vi "macro_Cmd_Follow_RamseteExecute.vi"() -> ()   [LabVIEW 2019, in "PathPlanner24.lvlib"]
uses:
  PathPlanner24.lvlib
  <vilib>/Rock Robotics/WPI/ThirdParty/JAS_Junk/TrajLib/Trajectory_Library.lvlib
  <vilib>/Rock Robotics/WPI/ThirdParty/JAS_Junk/TrajLib/TypeDef/TRANSLATION2D.ctl
  <vilib>/Rock Robotics/WPI/ThirdParty/JAS_Junk/TrajLib/TypeDef/ROTATION2D.ctl
  <vilib>/Rock Robotics/WPI/ThirdParty/JAS_Junk/TrajLib/TypeDef/POSE2D.ctl
  TypeDef/PathPlannerPathConstraints.ctl
  TypeDef/PathPlannerRotationTarget.ctl
  TypeDef/PathPlannerConstraintsZone.ctl
  ENum/PathPlanner_CommandUtilType_ENUM.ctl
  TypeDef/PathPlannerCommandUtil.ctl
  TypeDef/PathPlannerEventMarker.ctl
  TypeDef/PathPlannerGoalEndState.ctl
  TypeDef/PathPlannerPathPoint.ctl
  TypeDef/PathPlannerPath.ctl
  <vilib>/Rock Robotics/WPI/ThirdParty/JAS_Junk/TrajLib/TypeDef/CHASSIS_SPEEDS.ctl
panel:
  out "Complete":bool
  in  "CurrentChassisSpeeds":T1 {"vOmega" format="%10.3f"; "vY" format="%10.3f"; "vX" format="%10.3f"}
  in  "PathPlannerPath":T2={"BezierPoints"=[], "PreviewStartingRotation"={"VALUE"=0.0, "COS"=1.0, "SIN"=0.0}, "Reversed"=FALSE, "RotationTargets"=[], "ConstraintZones"=[], "EventMarkers"=[], "GlobalConstraints"={"MaxVelocityMps;"=0.0, "MaxAccelerationMpsSq;"=0.0, "MaxAngularVelRadPsEc;"=0.0, "MaxAngularAccRadPSecSq"=0.0, "Exists"=FALSE, "Unlimited"=FALSE, "NominalVoltageVolts"=12.0}, "GoalEndState"={"VelocityMPS"=0.0, "Rotation"={"VALUE"=0.0, "COS"=1.0, "SIN"=0.0}}, "AllPoints"=[]} {"AllPoints"."HolonomicRotation"."SIN" format="%13.4f"; "AllPoints"."HolonomicRotation"."COS" format="%13.4f"; "AllPoints"."HolonomicRotation"."VALUE" format="%13.4f"; "AllPoints"."Position"."Y" format="%14.3f"; "AllPoints"."Position"."X" format="%14.3f"; "GoalEndState"."Rotation"."SIN" format="%13.4f"; "GoalEndState"."Rotation"."COS" format="%13.4f"; "GoalEndState"."Rotation"."VALUE" format="%13.4f"; "RotationTargets"."rotation"."SIN" format="%13.4f"; "RotationTargets"."rotation"."COS" format="%13.4f"; "RotationTargets"."rotation"."VALUE" format="%13.4f"; "PreviewStartingRotation"."SIN" format="%13.4f"; "PreviewStartingRotation"."COS" format="%13.4f"; "PreviewStartingRotation"."VALUE" format="%13.4f"; "BezierPoints"."Y" format="%14.3f"; "BezierPoints"."X" format="%14.3f"}
  out "Left Speed Dmd M/S":dbl
  out "Right Speed Dmd M/S":dbl
  in  "Reset":bool
  in  "currentPose":T13={"TRANSLATION"={"X"=0.0, "Y"=0.0}, "ROTATION"={"VALUE"=0.0, "COS"=1.0, "SIN"=0.0}} {"ROTATION"."SIN" format="%13.4f"; "ROTATION"."COS" format="%13.4f"; "ROTATION"."VALUE" format="%13.4f"; "TRANSLATION"."Y" format="%14.3f"; "TRANSLATION"."X" format="%14.3f"}
  out "Position Error M":dbl
  out "At Reference":bool
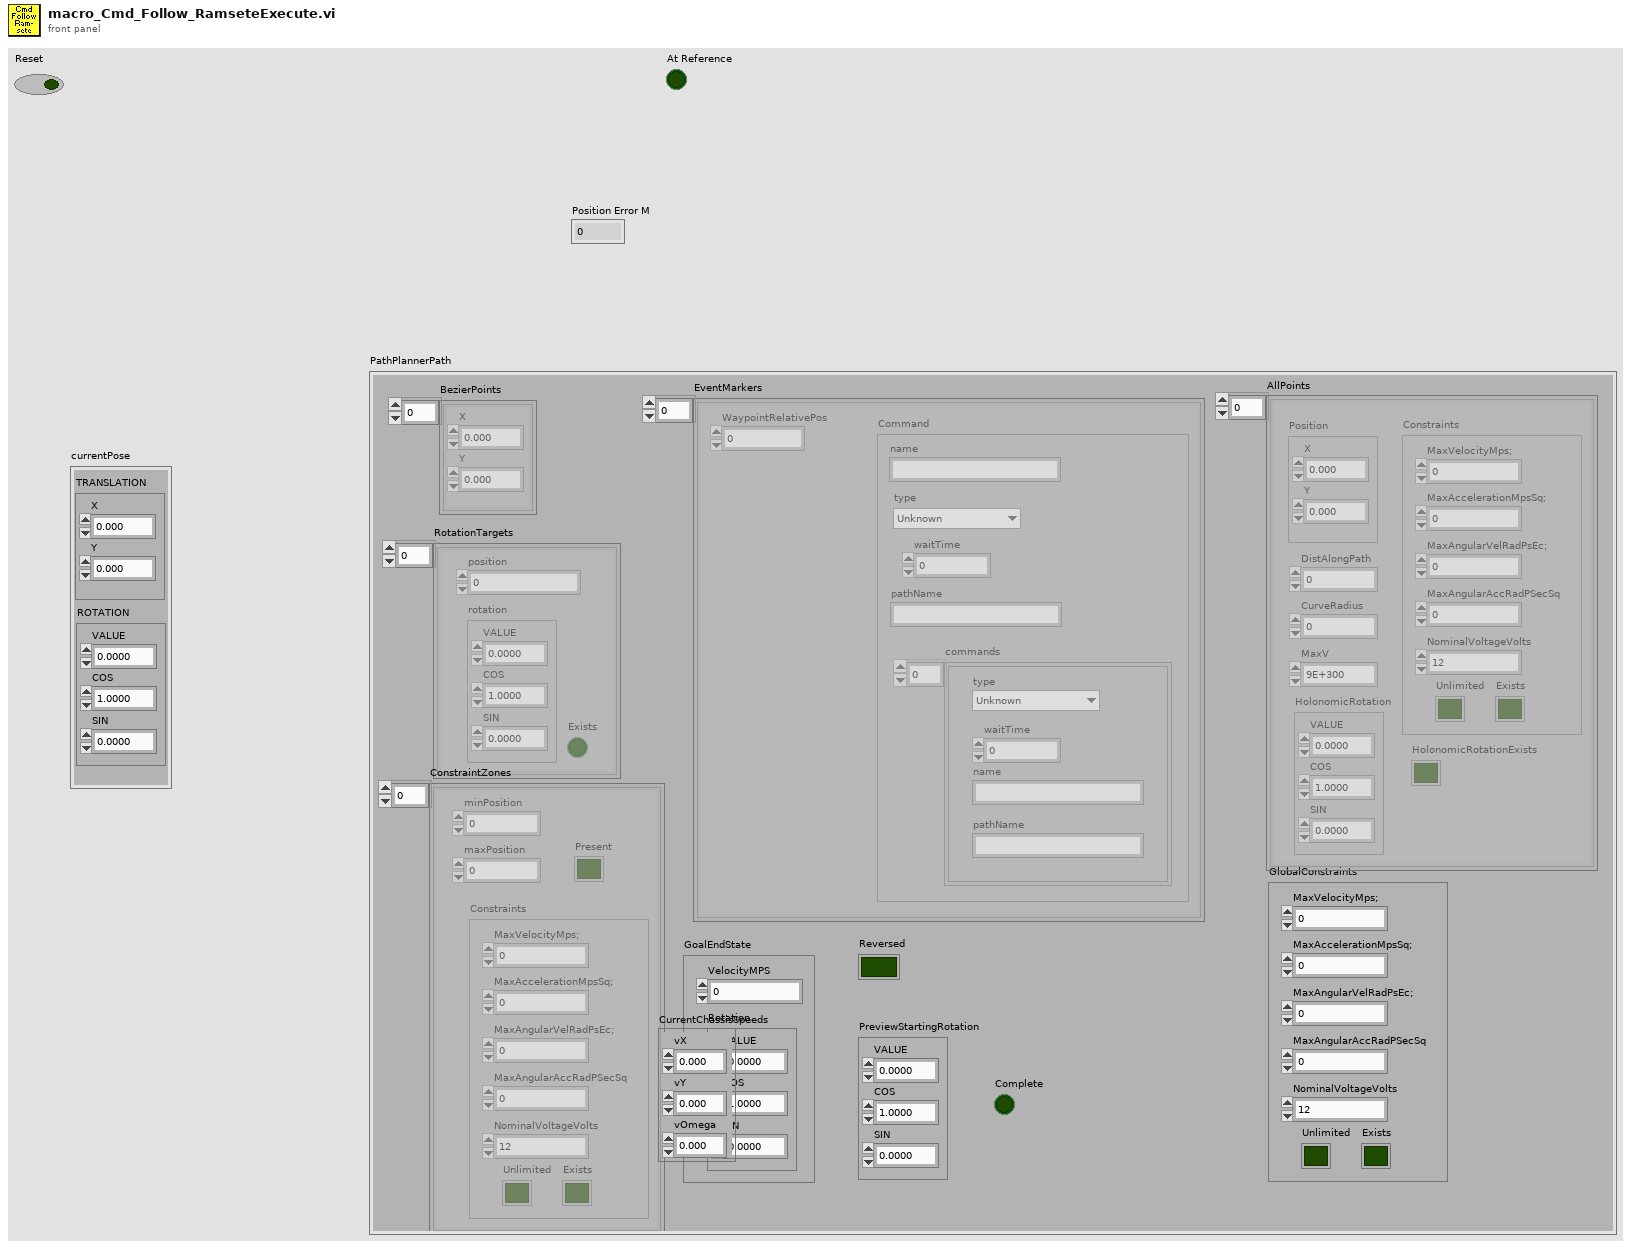
[diagram p1: front panel]
types:
  T1 = typedef "Trajectory_Library.lvlib/CHASSIS_SPEEDS.ctl" = cluster{"vX":dbl, "vY":dbl, "vOmega":dbl}
  T2 = typedef "PathPlanner24.lvlib/PathPlannerPath.ctl" = cluster{"BezierPoints":T3[], "PreviewStartingRotation":T4, "Reversed":bool, "RotationTargets":T5[], "ConstraintZones":T6[], "EventMarkers":T8[], "GlobalConstraints":T7, "GoalEndState":T11, "AllPoints":T12[]}
  T3 = typedef "Trajectory_Library.lvlib/TRANSLATION2D.ctl" = cluster{"X":dbl, "Y":dbl}
  T4 = typedef "Trajectory_Library.lvlib/ROTATION2D.ctl" = cluster{"VALUE":dbl, "COS":dbl, "SIN":dbl}
  T5 = typedef "PathPlanner24.lvlib/PathPlannerRotationTarget.ctl" = cluster{"rotation":T4, "position":dbl, "Exists":bool}
  T6 = typedef "PathPlanner24.lvlib/PathPlannerConstraintsZone.ctl" = cluster{"minPosition":dbl, "maxPosition":dbl, "Constraints":T7, "Present":bool}
  T7 = typedef "PathPlanner24.lvlib/PathPlannerPathConstraints.ctl" = cluster{"MaxVelocityMps;":dbl, "MaxAccelerationMpsSq;":dbl, "MaxAngularVelRadPsEc;":dbl, "MaxAngularAccRadPSecSq":dbl, "Exists":bool, "Unlimited":bool, "NominalVoltageVolts":dbl}
  T8 = typedef "PathPlanner24.lvlib/PathPlannerEventMarker.ctl" = cluster{"WaypointRelativePos":dbl, "Command":T9}
  T9 = typedef "PathPlanner24.lvlib/PathPlannerCommandUtil.ctl" = cluster{"waitTime":dbl, "name":string, "pathName":string, "commands":cluster{"type":T10, "waitTime":dbl, "name":string, "pathName":string}[], "type":T10}
  T10 = typedef "PathPlanner24.lvlib/PathPlanner_CommandUtilType_ENUM.ctl" = enum16{"Unknown", "Wait", "Named", "Path", "Sequential", "Parallel", "Race", "Deadline"}
  T11 = typedef "PathPlanner24.lvlib/PathPlannerGoalEndState.ctl" = cluster{"VelocityMPS":dbl, "Rotation":T4}
  T12 = typedef "PathPlanner24.lvlib/PathPlannerPathPoint.ctl" = cluster{"Position":T3, "HolonomicRotation":T4, "DistAlongPath":dbl, "CurveRadius":dbl, "MaxV":dbl, "Constraints":T7, "HolonomicRotationExists":bool}
  T13 = typedef "Trajectory_Library.lvlib/POSE2D.ctl" = cluster{"TRANSLATION":T3, "ROTATION":T4}
  T14 = typedef "PathPlanner24.lvlib/PathPlannerReplanningConfig.ctl" = cluster{"enableInitialReplanning":bool, "enableDynamicReplanning":bool, "dynamicReplanningTotalErrorThreshold":dbl, "dynamicReplanningErrorSpikeThreshold":dbl}
  T15 = typedef "Trajectory_Library.lvlib/RAMSETE_EXE_TUNING.ctl" = cluster{"B":dbl, "Zeta":dbl, "X Tolerance M":dbl, "Y Tolerance M":dbl, "Heading Tolerance RAD":dbl, "Track Width M":dbl, "Max Speed M/S":dbl}
  T16 = typedef "PathPlanner24.lvlib/PathPlannerCmdFollowRamConfig.ctl" = cluster{"ControlPastEnd_Sec":dbl, "ReplanningConfig":T14, "Trigger Events":bool, "RAMSETE_EXE_TUNING SI":T15}
  T17 = cluster{"Left Speed Dmd M/S":dbl, "Right Speed Dmd M/S":dbl}
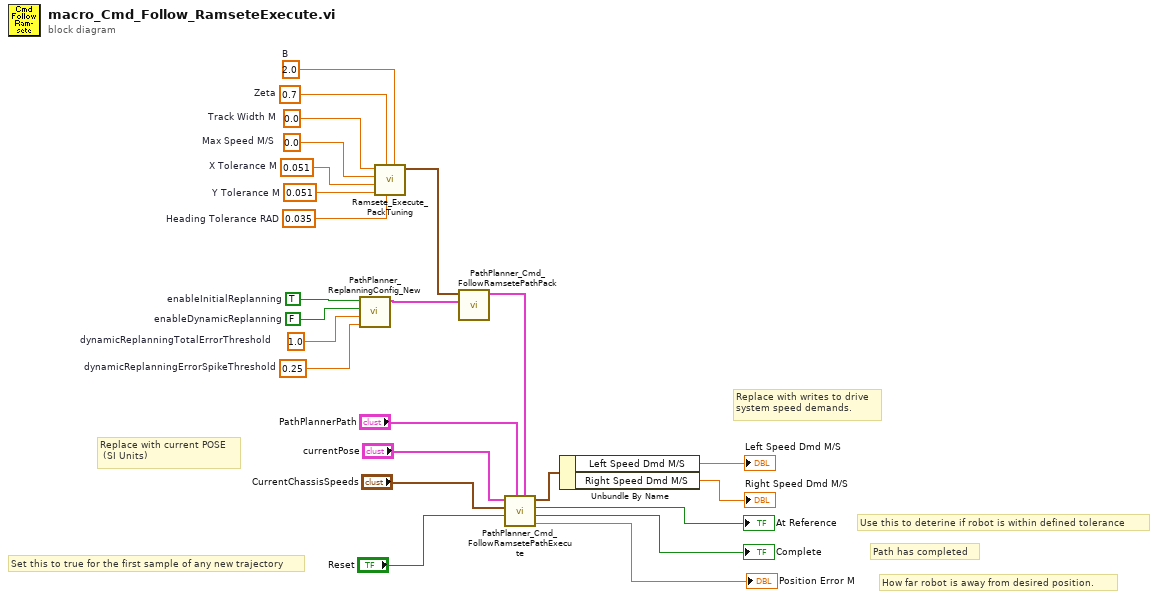
[diagram p0: block diagram]
diagram:
  w13 = TRUE  # enableInitialReplanning
  w14 = FALSE  # enableDynamicReplanning
  w15 = 1.0  # dynamicReplanningTotalErrorThreshold
  w16 = 0.25  # dynamicReplanningErrorSpikeThreshold
  w24 = 0.0  # Track Width M
  w23 = 0.0  # Max Speed M/S
  w22 = 0.051  # X Tolerance M
  w21 = 0.051  # Y Tolerance M
  w20 = 0.7  # Zeta
  w19 = 0.035  # Heading Tolerance RAD
  w18 = 2.0  # B
  # "Path has completed"
  # "Replace with writes to drive\nsystem speed demands."
  # "Replace with current POSE\n (SI Units)"
  # "How far robot is away from desired position."
  # "Use this to deterine if robot is within defined tolerance"
  # "Set this to true for the first sample of any new trajectory"
  n1 = call "PathPlanner_ReplanningConfig_New.vi"("dynamicReplanningErrorSpikeThreshold"=w16, "dynamicReplanningTotalErrorThreshold"=w15, "enableDynamicReplanning"=w14, "enableInitialReplanning"=w13) -> ("ReplanningConfig"=w12:T14)  [unwired: 7 in]
  n2 = call <vilib>:"Ramsete_Execute_PackTuning.vi"("B"=w18, "Heading Tolerance RAD"=w19, "Zeta"=w20, "Y Tolerance M"=w21, "X Tolerance M"=w22, "Max Speed M/S"=w23, "Track Width M"=w24) -> ("RAMSETE_EXE_TUNING"=w11:T15)  [unwired: 4 in]
  n3 = call "PathPlanner_Cmd_FollowRamsetePathPack.vi"("ReplanningConfig"=w12, "RAMSETE_EXE_TUNING"=w11) -> ("PathPlanner_Ctrl_RamDrvConfig"=w17:T16)  [unwired: 9 in]
  n4 = call "PathPlanner_Cmd_FollowRamsetePathExecute.vi"("PathPlanner_Cmd_FollowRamConfig"=w17, "PathPlannerPath"="PathPlannerPath", "Reset"="Reset", "CurrentChassisSpeeds"="CurrentChassisSpeeds", "Current Pose SI"="currentPose") -> ("Position Error M"=→"Position Error M":dbl, "Complete"=→"Complete":bool, "At Reference"=→"At Reference":bool, "Left Right Speed Dmds"=w6:T17)  [unwired: 2 in, 1 out]
  n5 = Unbundle By Name(w6) -> ("Left Speed Dmd M/S"=→"Left Speed Dmd M/S":dbl, "Right Speed Dmd M/S"=→"Right Speed Dmd M/S":dbl)
